vi "ActOnResult.vi"(0 "object in":refnum<class "ExtraGUI.lvclass">, 1 "Data":variant, 5 "error in (no error)":errorcluster) -> (14 "object out":refnum<class "ExtraGUI.lvclass">, 19 "error out":errorcluster)   [LabVIEW 2017, in "ExtraGUI.lvclass"]
uses:
  ExtraGUI.lvclass
  ExtraGUI.lvclass/ExtraGUI.ctl
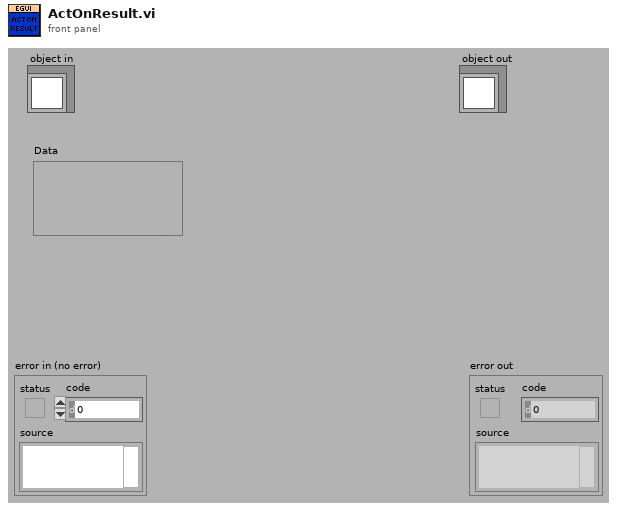
[diagram p1: front panel]
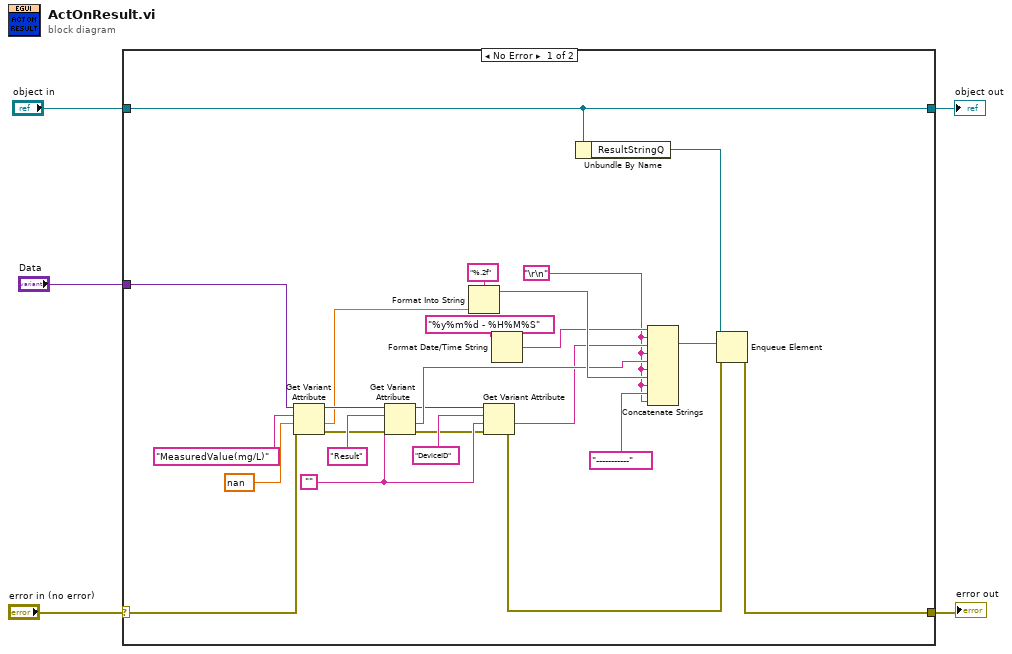
[diagram p0: block diagram]
diagram:
  n1 = case shown="No Error" "error in (no error)" {
    selector: "error in (no error)" -> [w11 w32]
    tunnel: [w28 w32] -> w4
    tunnel: [w30 w31] -> w2
    tunnel: "object in" -> [w30 w31]
    tunnel: "Data" -> [w8 _]
    frame No Error {
      w6 = "\r\n" ("format string")
      w19 = ""
      n2 = Get Variant Attribute(Variant=w8, name="MeasuredValue(mg/L)", default value (empty Variant)=nan, error in=w11) -> (duplicate Variant=w22:variant, value=w17:dbl, error out=w20:errorcluster)  [unwired: 1 out]
      n3 = Get Variant Attribute(Variant=w22, name="Result", default value (empty Variant)=w19, error in=w20) -> (duplicate Variant=w12:variant, value=w16:string, error out=w13:errorcluster)  [unwired: 1 out]
      n4 = Format Into String(format string="%.2f", w17) -> (resulting string=w25:string)  [unwired: 2 in, 1 out]
      n5 = Get Variant Attribute(Variant=w12, name="DeviceID", default value (empty Variant)=w19, error in=w13) -> (value=w14:string, error out=w10:errorcluster)  [unwired: 2 out]
      n6 = Format Date/Time String(time format string (%c)="%y%m%d - %H%M%S") -> (date/time string=w15:string)  [unwired: 1 in, 1 out]
      n7 = Unbundle By Name(w30) -> ("ResultStringQ"=w29:refnum<queue>)
      n8 = Concatenate Strings(w15, w6, w14, w6, w16, w6, w25, w6, "-----------" ("format string"), w6) -> (w9:string)
      n9 = Enqueue Element(queue=w29, element=w9, error in (no error)=w10) -> (error out=w28:errorcluster)  [unwired: 1 in, 2 out]
    }
    frame Error {
    }
  }
  "error out" <- w4
  "object out" <- w2
